vi "Init.vi"(10 "Queue":refnum<class "Queue.lvclass">) -> (3 "Last Ack Created Queue Msg Strategy out":refnum<class "Last Ack Created Queue Msg Strategy.lvclass">)   [LabVIEW 2021, in "jettl.lvlib" / "Last Ack Created Queue Msg Strategy.lvlib" / "Last Ack Created Queue Msg Strategy.lvclass"]
uses:
  Last Ack Created Queue Msg Strategy.lvclass
  Queue/Queue.lvclass
  Last Ack Created Queue Msg Strategy.lvclass/Last Ack Created Queue Msg Strategy.ctl
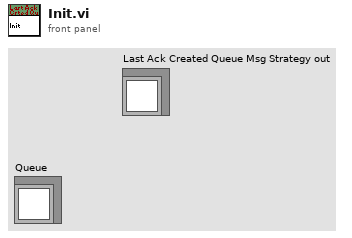
[diagram p1: front panel]
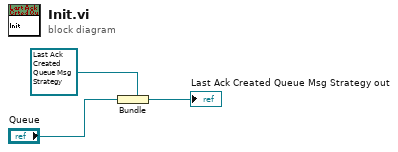
[diagram p0: block diagram]
diagram:
  n1 = Bundle "Bundle"(cluster=refnum<class "Last Ack Created Queue Msg Strategy.lvclass"> refnum ("Last Ack Msg in"), "Queue") -> (→"Last Ack Created Queue Msg Strategy out":refnum<class "Last Ack Created Queue Msg Strategy.lvclass">)
